vi "Scan.vi"() -> (0 "Error Out":errorcluster caption="错误输出", 3 "Barcode":string caption="扫描条码/Barcode")   [LabVIEW 2017]
uses:
  <vilib>/Instr/_visa.llb/VISA Configure Serial Port (Instr).vi
panel:
  in  "Exit":bool
  # "手动扫描"
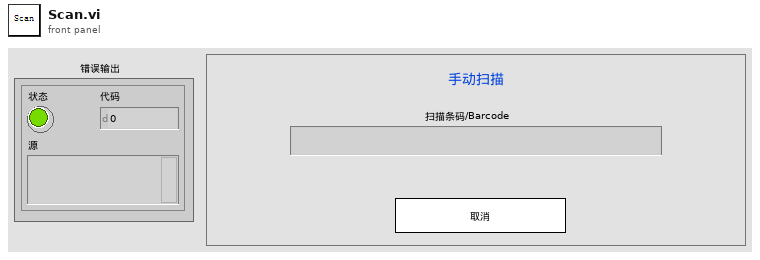
[diagram p1: front panel]
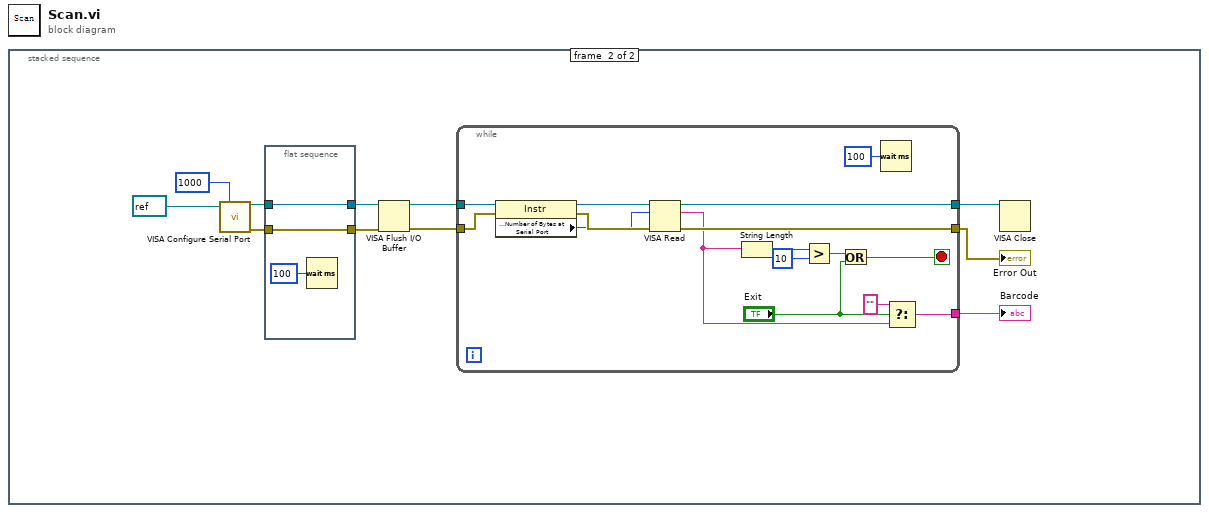
[diagram p0: block diagram]
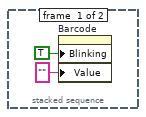
[diagram p2: hidden frame]
diagram:
  n1 = stacked-sequence {
    frame #0 {
      n2 = property on="Barcode" class="Str"("Blinking"=TRUE, "Value"="" ("Barcode")) -> ()  [unwired: 2 in, 2 out]
    }
    frame #1 {
      n3 = call-poly "VISA Configure Serial Port"("VISA resource name"=refnum<visa-resource-name> refnum, "timeout (10sec)"=u32 1000) -> ("VISA resource name out"=w11:refnum<visa-resource-name>, "error out"=w12:errorcluster)  [unwired: 12 in]
      n4 = flat-sequence {
        tunnel: w12 -> [w14]
        tunnel: w11 -> [w15]
        tunnel: [w15] -> w10
        tunnel: [w14] -> w9
        frame #0 {
          n5 = Wait (ms)(milliseconds to wait=u32 100) -> ()  [unwired: 1 out]
        }
      }
      n6 = VISA Flush I/O Buffer(VISA resource name=w10, error in (no error)=w9) -> (VISA resource name out=w8:refnum<visa-resource-name>, error out=w7:errorcluster)  [unwired: 1 in]
      n7 = while {
        tunnel: w8 -> [w32]
        tunnel: w7 -> [w31]
        tunnel: [w27] -> w6
        tunnel: [w26] -> w4
        tunnel: [w20] -> w5
        stop <- w22 stop-if-true
        n8 = property class="Instr"(reference=w32, error in=w31) -> (reference out=w30:refnum<visa-resource-name>, error out=w29:errorcluster, "Serial Settings:Number of Bytes at Serial Port"=w28:u32)
        n9 = VISA Read(VISA resource name=w30, byte count=w28, error in (no error)=w29) -> (VISA resource name out=w27:refnum<visa-resource-name>, read buffer=w17:string, error out=w26:errorcluster)  [unwired: 1 out]
        n10 = String Length(string=w17) -> (length=w25:i32)
        n11 = Greater?(x=w25, y=10) -> (0:w23:bool)
        n12 = Or(x=w23, y="Exit") -> (x .or. y?=w22:bool)
        n13 = Wait (ms)(milliseconds to wait=u32 100) -> ()  [unwired: 1 out]
        n14 = Select(t="", s="Exit", f=w17) -> (s? t:f=w20:string)
      }
      "Barcode" <- w5
      "Error Out" <- w4
      n15 = VISA Close(VISA resource name=w6) -> ()  [unwired: 1 in, 1 out]
    }
  }
